vi "Spätzle_Control.vi"() -> ()   [LabVIEW 2014]
doc: "Mit diesem VI wird eine Autowäsche simuliert. Mit den Waschprogrammelementen wählen Sie die gewünschten Optionen aus. Wenn keine Option ausgewählt wird, ist die Hochdruckreinigung das Standardwaschprogramm. Nach Klick auf \"Start\" beginnt die Wäsche. Mit dem Element \"Schieberegler für Fahrzeugposition\" wird die Position des Fahrzeugs simuliert. Wenn sich das Fahrzeug in der falschen Position für das aktuelle Programm befindet, leuchtet die entsprechende Anzeige und das Fahrzeug muss bewegt werden. Die Anzeige der Waschanlage stellt den aktuellen Status des Waschprogramms dar. Mit der Schaltfläche \"Programm stoppen\" wird die Autowaschanlage sofort gestoppt."
uses:
  Controls/Options.ctl
  Controls/Simulation Position Control.ctl
  Controls/Indicators.ctl
  Controls/State Control Enum.ctl
panel:
  in  "Stopp":bool
  out "Time (s)":dbl format="%#.2g"
  out "Anzeigen der Waschanlage":T1
  in  "Plate Position":T2 scale=0.0..4.0
  out "Availability":bool
  in  "Start":bool
  in  "Optional Toppings":T3
  # "User Options"
  # "Machine Status"
  # "Simulation for Position"
  # "Use the slider to simulate the position of the transport system.\nThe slider has to be in the right position for each state to proceed."
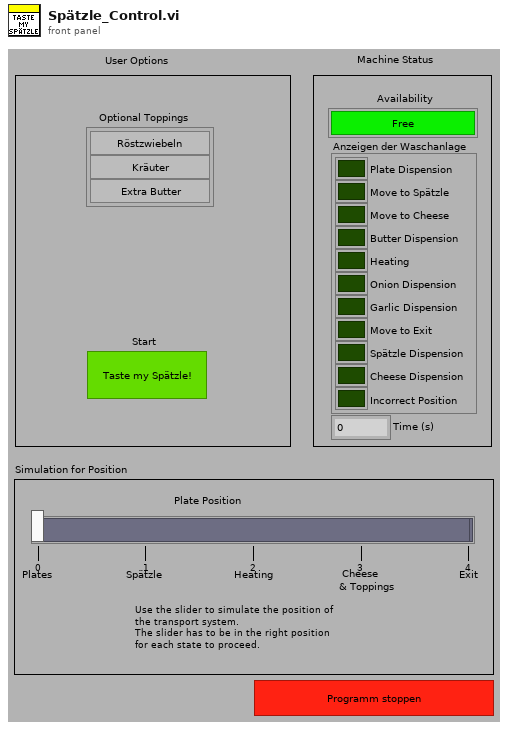
[diagram p1: front panel]
types:
  T1 = typedef "Indicators.ctl" = cluster{"Plate Dispension":bool, "Move to Spätzle":bool, "Move to Cheese":bool, "Butter Dispension":bool, "Heating":bool, "Onion Dispension":bool, "Garlic Dispension":bool, "Move to Exit":bool, "Spätzle Dispension":bool, "Cheese Dispension":bool, "Incorrect Position":bool}
  T2 = typedef "Simulation Position Control.ctl" = i32
  T3 = typedef "Options.ctl" = cluster{"Röstzwiebeln":bool, "Kräuter":bool, "Extra Butter":bool}
  T4 = typedef "State Control Enum.ctl" = enum16{"Initialize", "Wait for Start", "Plate Dispension", "Spätzle Dispension", "Heating", "Cheese Dispension", "Onion Dispension", "Garlic Dispension", "Butter Dispension", "Move to Spätzle", "Move To Cheese", "Move to Exit", "Stop", "Skip"}
  T5 = enum8{"Enabled", "Disabled", "Disabled and Grayed Out"}
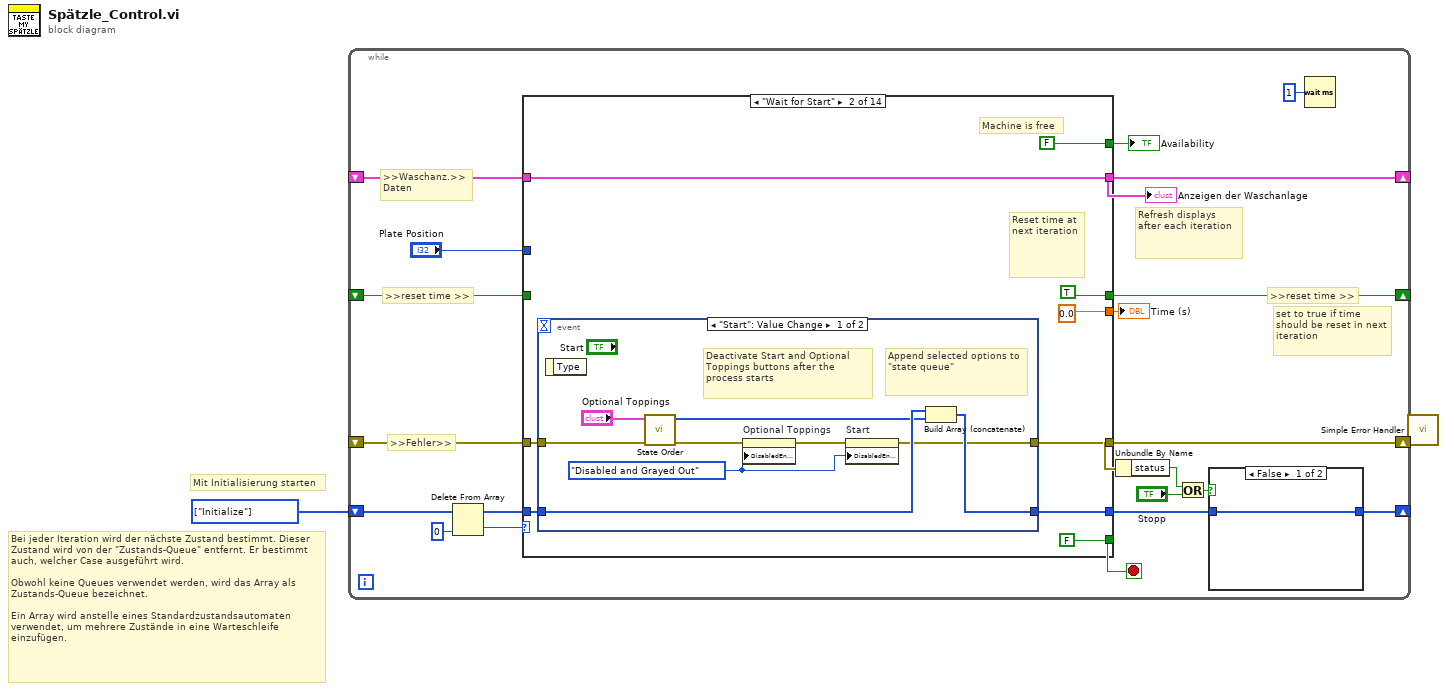
[diagram p0: block diagram]
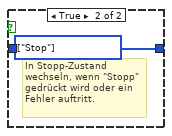
[diagram p2: hidden frame]
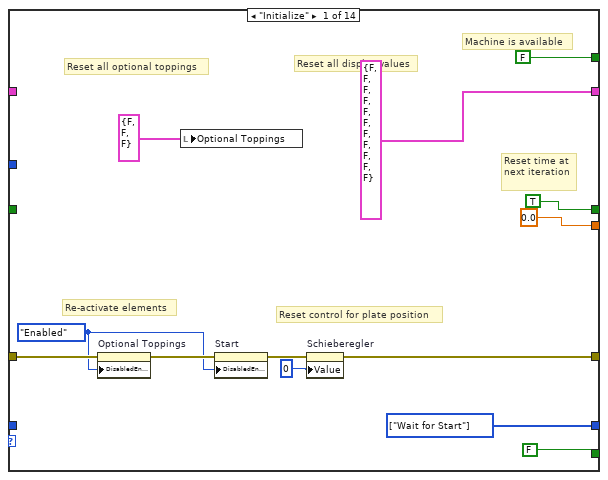
[diagram p3: hidden frame]
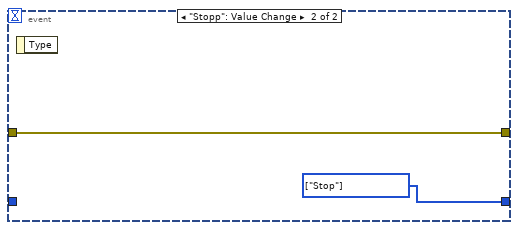
[diagram p4: hidden frame]
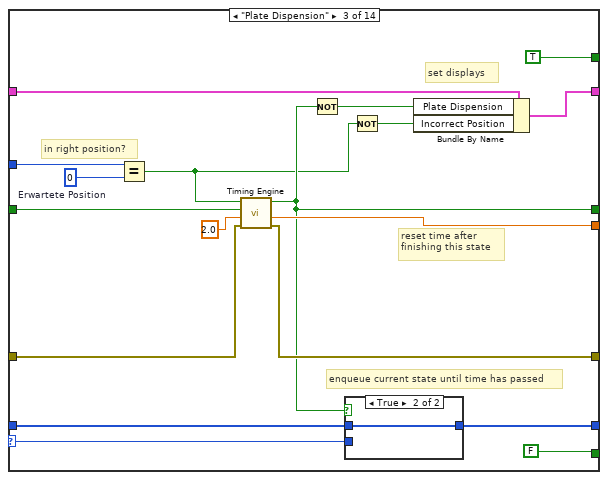
[diagram p5: hidden frame]
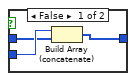
[diagram p6: hidden frame]
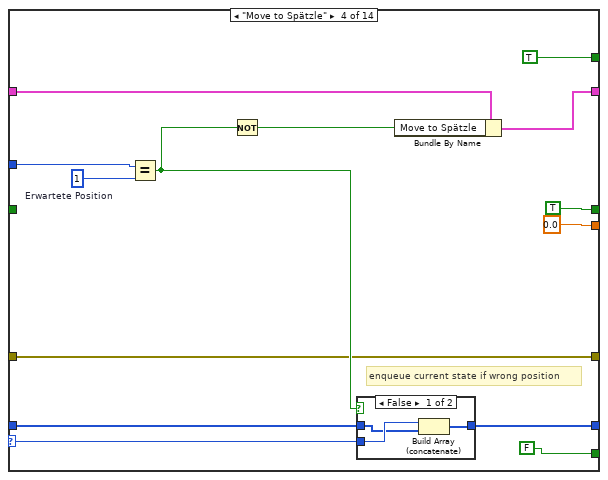
[diagram p7: hidden frame]
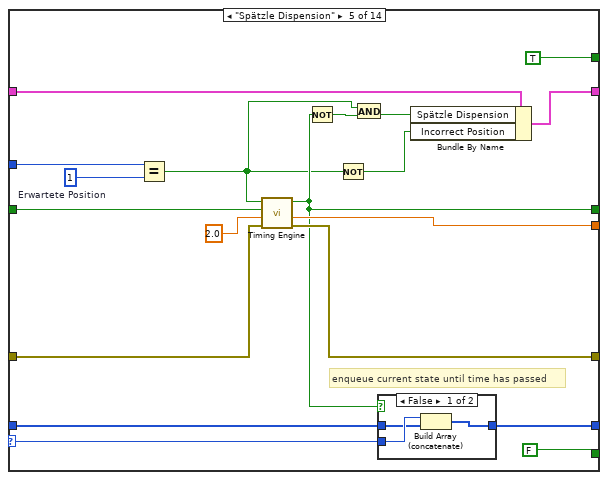
[diagram p9: hidden frame]
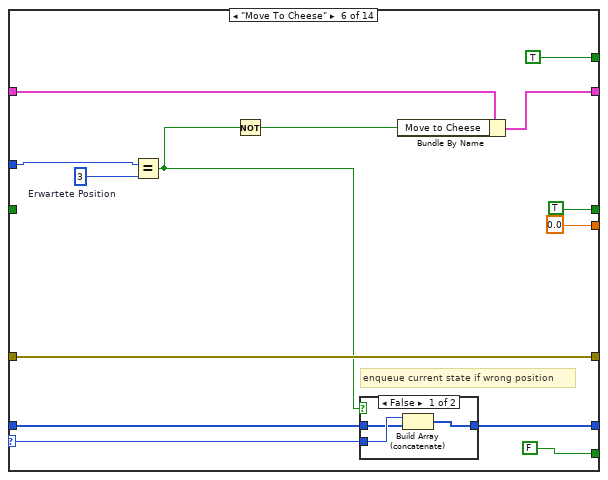
[diagram p11: hidden frame]
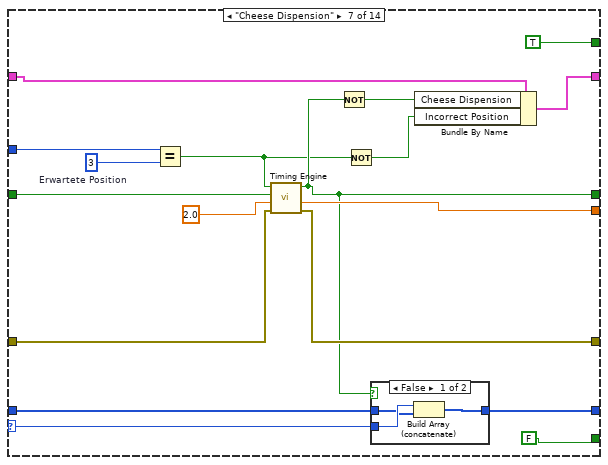
[diagram p13: hidden frame]
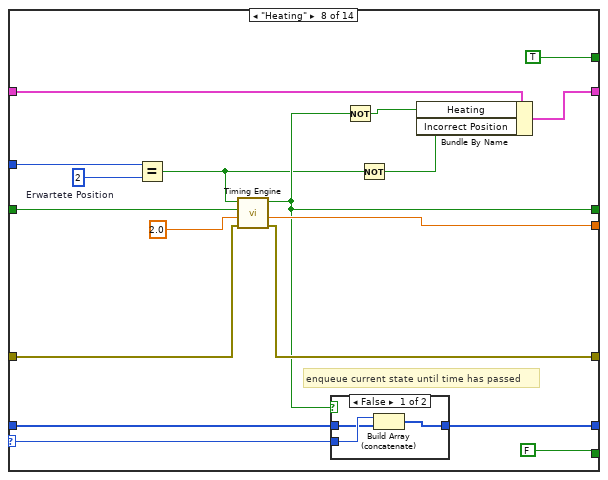
[diagram p15: hidden frame]
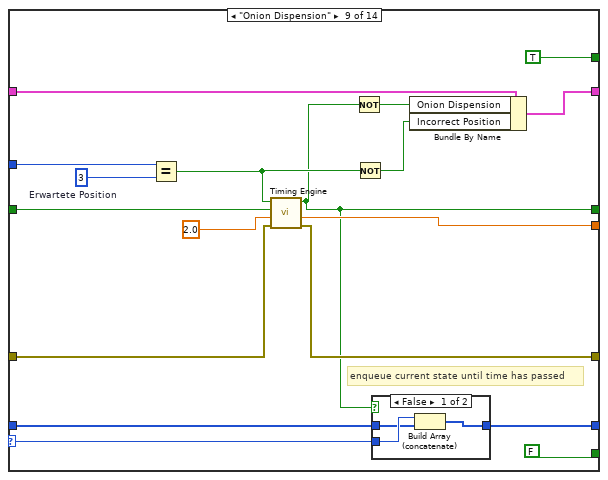
[diagram p17: hidden frame]
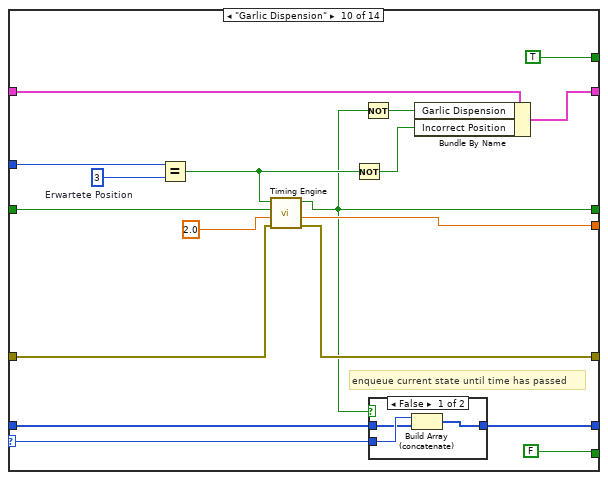
[diagram p19: hidden frame]
diagram:
  w2 = T4[] [enum."Initialize"] items=["Initialize", "Wait for Start", "Plate Dispension", "Spätzle Dispension", "Heating", "Cheese Dispension", "Onion Dispension", "Garlic Dispension", "Butter Dispension", "Move to Spätzle", "Move To Cheese", "Move to Exit", "Stop", "Skip"]
  # "Mit Initialisierung starten"
  # "Bei jeder Iteration wird der nächste Zustand bestimmt. Dieser Zustand wird von der \"Zustands-Queue\" entfernt. Er bestimmt auch, welcher Case ausgeführt wird. \n\nObwohl keine Queues verwendet werden, wird das Array als Zustands-Queue bezeichnet.  \n\nEin Array wird anstelle eines Standardzustandsautomaten verwendet, um mehrere Zustände in eine Warteschleife einzufügen."
  n1 = while "While-Schleife" {
    shift-right: [w15] -> _
    shift-left: w2 -> [w3]
    shift-right: [w18] -> _
    shift-left: _ -> [w19]
    shift-right: [w7] -> w1
    shift-left: _ -> [w14]
    shift-right: [w13] -> _
    shift-left: _ -> [w12]
    stop <- w9 stop-if-true
    # "Refresh displays after each iteration"
    # "set to true if time should be reset in next iteration"
    # ">>reset time >>"
    # ">>Fehler>>"
    # ">>Waschanz.>>\nDaten"
    # ">>reset time >>"
    n2 = Delete From Array ("Aus Array entfernen")(array=w3, index=0 ("Index")) -> (deleted portion=w20:T4, array with subset deleted=w21:T4[])  [unwired: 1 in]
    n3 = case "Case-Struktur" shown="\"Wait for Start\"" w20 {
      selector: w20 -> [_ _ w64 w83 w107 w124 w154 w170 w191 w219 w234 _ _ _]
      tunnel: w21 -> [_ w44 w63 w84 w108 w125 w153 w171 w190 w218 w233 w250 _ _]
      tunnel: [w29 w45 w65 w85 w106 w123 w152 w169 w189 w211 w235 w250 w262 w273] -> w16
      tunnel: [T1 {"Plate Dispension"=FALSE, "Move to Spätzle"=FALSE, "Move to Cheese"=FALSE, "Butter Dispension"=FALSE, "Heating"=FALSE, "Onion Dispension"=FALSE, "Garlic Dispension"=FALSE, "Move to Exit"=FALSE, "Spätzle Dispension"=FALSE, "Cheese Dispension"=FALSE, "Incorrect Position"=FALSE} ("Anzeigen der Waschanlage 2") w38 w66 w88 w109 w133 w146 w172 w192 w215 w236 w255 w266 T1 {"Plate Dispension"=FALSE, "Move to Spätzle"=FALSE, "Move to Cheese"=FALSE, "Butter Dispension"=FALSE, "Heating"=FALSE, "Onion Dispension"=FALSE, "Garlic Dispension"=FALSE, "Move to Exit"=FALSE, "Spätzle Dispension"=FALSE, "Cheese Dispension"=FALSE, "Incorrect Position"=FALSE} ("Anzeigen der Waschanlage 2")] -> w18
      tunnel: w19 -> [_ w38 w67 w89 w110 w134 w147 w173 w193 w216 w237 w255 w265 _]
      tunnel: [FALSE ("Einfahrt") FALSE ("Einfahrt") TRUE ("Einfahrt") TRUE ("Einfahrt") TRUE ("Einfahrt") TRUE ("Einfahrt") TRUE ("Einfahrt") TRUE ("Einfahrt") TRUE ("Einfahrt") TRUE ("Einfahrt") TRUE ("Einfahrt") TRUE ("Einfahrt") TRUE ("Einfahrt") FALSE ("Einfahrt")] -> w17
      tunnel: w14 -> [w35 w43 w71 w80 w112 w129 w150 w166 w197 w212 w242 w251 w261 w280]
      tunnel: [w25 w42 w72 w80 w111 w129 w151 w167 w196 w220 w241 w252 w261 w279] -> w7
      tunnel: [TRUE ("Zeit abgelaufen?") TRUE ("Einfahrt") w61 TRUE ("Zeit abgelaufen?") w103 TRUE ("Zeit abgelaufen?") w142 w164 w184 w206 w230 w254 TRUE ("Zeit abgelaufen?") TRUE ("Zeit abgelaufen?")] -> w13
      tunnel: w12 -> [_ _ w74 _ w113 _ w149 w175 w194 w213 w240 w254 _ _]
      tunnel: [0.0 ("Verstrichene Zeit") 0.0 ("Verstrichene Zeit") w73 0.0 ("Verstrichene Zeit") w104 0.0 ("Verstrichene Zeit") w145 w174 w198 w217 w238 w253 0.0 ("Verstrichene Zeit") 0.0 ("Verstrichene Zeit")] -> w11
      tunnel: "Plate Position" -> [_ _ w69 w90 w114 w127 w148 w176 w195 w214 w239 _ w268 _]
      tunnel: [FALSE ("Einfahrt") FALSE ("Einfahrt") FALSE ("Einfahrt") FALSE ("Einfahrt") FALSE ("Einfahrt") FALSE ("Einfahrt") FALSE ("Einfahrt") FALSE ("Einfahrt") FALSE ("Einfahrt") FALSE ("Einfahrt") FALSE ("Einfahrt") FALSE ("Einfahrt") FALSE ("Einfahrt") TRUE ("Einfahrt")] -> w9
      frame "Initialize" {
        w29 = T4[] [enum."Wait for Start"] items=["Initialize", "Wait for Start", "Plate Dispension", "Spätzle Dispension", "Heating", "Cheese Dispension", "Onion Dispension", "Garlic Dispension", "Butter Dispension", "Move to Spätzle", "Move To Cheese", "Move to Exit", "Stop", "Skip"]
        w26 = T5."Enabled" ("Deaktiviert")
        # "Reset time at next iteration"
        # "Re-activate elements"
        # "Reset control for plate position"
        # "Machine is available"
        # "Reset all display values"
        # "Reset all optional toppings"
        n4 = property on="Optional Toppings" class="Clust (strict)"(error in=w35, "DisabledEnum"=w26) -> (error out=w34:errorcluster)  [unwired: 1 in, 1 out]
        n5 = local write "Optional Toppings"(T3 {"Röstzwiebeln"=FALSE, "Kräuter"=FALSE, "Extra Butter"=FALSE} ("Waschprogramme")) -> ()
        n6 = property on="Start" class="Bool"(error in=w34, "DisabledEnum"=w26) -> (error out=w28:errorcluster)  [unwired: 1 in, 1 out]
        n7 = property on="Schieberegler" class="Slide (strict)"(error in=w28, "Value"=0) -> (error out=w25:errorcluster)  [unwired: 1 in, 1 out]
      }
      frame "Wait for Start" {
        # "Reset time at next iteration"
        # "Machine is free"
        n8 = event shown="[0] \"Start\": Value Change" {
          selector: _ -> [_ _]
          dyn-events: _ -> [_ _]
          timeout: _ -> [_ _]
          tunnel: [w51 w57] -> w45
          tunnel: w44 -> [w53 _]
          tunnel: [w47 w56] -> w42
          tunnel: w43 -> [w48 w56]
          event "Start": Value Change {
            w49 = T5."Disabled and Grayed Out" ("Deaktiviert")
            # "Append selected options to \"state queue\""
            # "Deactivate Start and Optional Toppings buttons after the process starts"
            n9 = event-data ("Ereignisdatenknoten")() -> ()  [unwired: 2 out]
            n10 = call "State Order.vi"("Fehler (Eingang)"=w48, "Options"="Optional Toppings") -> ("Fehler (Ausgang)"=w54:errorcluster, "States"=w52:T4[])  [unwired: 8 out]
            n11 = property on="Optional Toppings" class="Clust (strict)"(error in=w54, "DisabledEnum"=w49) -> (error out=w50:errorcluster)  [unwired: 1 in, 1 out]
            n12 = property on="Start" class="Bool"(error in=w50, "DisabledEnum"=w49) -> (error out=w47:errorcluster)  [unwired: 1 in, 1 out]
            n13 = Build Array (concatenate) ("Array erstellen")(w53, w52) -> (w51:T4[])
          }
          event "Stopp": Value Change {
            w57 = T4[] [enum."Stop"] items=["Initialize", "Wait for Start", "Plate Dispension", "Spätzle Dispension", "Heating", "Cheese Dispension", "Onion Dispension", "Garlic Dispension", "Butter Dispension", "Move to Spätzle", "Move To Cheese", "Move to Exit", "Stop", "Skip"]
            n14 = event-data ("Ereignisdatenknoten")() -> ()  [unwired: 2 out]
          }
        }
      }
      frame "Plate Dispension" {
        w68 = T2 0  # Erwartete Position
        # "in right position?"
        # "enqueue current state until time has passed"
        # "reset time after finishing this state"
        # "set displays"
        n15 = Equal? ("Gleich?")(x=w69, y=w68) -> (x = y?=w59:bool)
        n16 = call "Timing Engine.vi"("Fehler (Eingang)"=w71, "Zeitbegrenzung"=2.0 ("Waschzykluszeit"), "Zurücksetzen"=w74, "Zeitfortschritt?"=w59) -> ("Fehler (Ausgang)"=w72:errorcluster, "Verstrichene Zeit"=w73:dbl, "Zeit abgelaufen?"=w61:bool)  [unwired: 5 out]
        n17 = Not ("NICHT")(x=w61) -> (.not. x?=w60:bool)
        n18 = case shown="True" w61 {
          tunnel: [w78 w79] -> w65
          tunnel: w64 -> [w77 _]
          tunnel: w63 -> [w76 w79]
          frame False {
            n19 = Build Array (concatenate) ("Array erstellen")(w77, w76) -> (w78:T4[])
          }
          frame True {
          }
        }
        n20 = Not(x=w59) -> (.not. x?=w58:bool)
        n21 = Bundle By Name ("Nach Namen bündeln")(cluster=w67, "Plate Dispension"=w60, "Incorrect Position"=w58) -> (w66:T1)
      }
      frame "Move to Spätzle" {
        w91 = T2 1  # Erwartete Position
        # "enqueue current state if wrong position"
        n22 = Equal?(x=w90, y=w91) -> (x = y?=w92:bool)
        n23 = Not(x=w92) -> (.not. x?=w93:bool)
        n24 = case shown="False" w92 {
          tunnel: [w94 w97] -> w85
          tunnel: w84 -> [w95 w97]
          tunnel: w83 -> [w96 _]
          frame False {
            n25 = Build Array (concatenate)(w96, w95) -> (w94:T4[])
          }
          frame True {
          }
        }
        n26 = Bundle By Name ("Nach Namen bündeln")(cluster=w89, "Move to Spätzle"=w93) -> (w88:T1)
      }
      frame "Spätzle Dispension" {
        w102 = T2 1  # Erwartete Position
        # "enqueue current state until time has passed"
        n27 = Equal? ("Gleich?")(x=w114, y=w102) -> (x = y?=w98:bool)
        n28 = call "Timing Engine.vi"("Fehler (Eingang)"=w112, "Zeitbegrenzung"=2.0 ("Waschzykluszeit"), "Zurücksetzen"=w113, "Zeitfortschritt?"=w98) -> ("Fehler (Ausgang)"=w111:errorcluster, "Verstrichene Zeit"=w104:dbl, "Zeit abgelaufen?"=w103:bool)  [unwired: 5 out]
        n29 = Not ("NICHT")(x=w103) -> (.not. x?=w101:bool)
        n30 = Not(x=w98) -> (.not. x?=w100:bool)
        n31 = And(x=w98, y=w101) -> (x .and. y?=w99:bool)
        n32 = case shown="False" w103 {
          tunnel: [w119 w120] -> w106
          tunnel: w107 -> [w118 _]
          tunnel: w108 -> [w117 w120]
          frame False {
            n33 = Build Array (concatenate) ("Array erstellen")(w118, w117) -> (w119:T4[])
          }
          frame True {
          }
        }
        n34 = Bundle By Name ("Nach Namen bündeln")(cluster=w110, "Spätzle Dispension"=w99, "Incorrect Position"=w100) -> (w109:T1)
      }
      frame "Move To Cheese" {
        w126 = T2 3  # Erwartete Position
        # "enqueue current state if wrong position"
        n35 = Equal?(x=w127, y=w126) -> (x = y?=w122:bool)
        n36 = Not(x=w122) -> (.not. x?=w121:bool)
        n37 = case shown="False" w122 {
          tunnel: [w137 w138] -> w123
          tunnel: w124 -> [w136 _]
          tunnel: w125 -> [w135 w138]
          frame False {
            n38 = Build Array (concatenate) ("Array erstellen")(w136, w135) -> (w137:T4[])
          }
          frame True {
          }
        }
        n39 = Bundle By Name ("Nach Namen bündeln")(cluster=w134, "Move to Cheese"=w121) -> (w133:T1)
      }
      frame "Cheese Dispension" {
        w143 = T2 3  # Erwartete Position
        n40 = Equal? ("Gleich?")(x=w148, y=w143) -> (x = y?=w141:bool)
        n41 = call "Timing Engine.vi"("Fehler (Eingang)"=w150, "Zeitbegrenzung"=2.0 ("Waschzykluszeit"), "Zurücksetzen"=w149, "Zeitfortschritt?"=w141) -> ("Fehler (Ausgang)"=w151:errorcluster, "Verstrichene Zeit"=w145:dbl, "Zeit abgelaufen?"=w142:bool)  [unwired: 5 out]
        n42 = Not(x=w142) -> (.not. x?=w139:bool)
        n43 = Not(x=w141) -> (.not. x?=w140:bool)
        n44 = case shown="False" w142 {
          tunnel: [w159 w160] -> w152
          tunnel: w154 -> [w158 _]
          tunnel: w153 -> [w157 w160]
          frame False {
            n45 = Build Array (concatenate) ("Array erstellen")(w158, w157) -> (w159:T4[])
          }
          frame True {
          }
        }
        n46 = Bundle By Name ("Nach Namen bündeln")(cluster=w147, "Cheese Dispension"=w139, "Incorrect Position"=w140) -> (w146:T1)
      }
      frame "Heating" {
        w165 = T2 2  # Erwartete Position
        # "enqueue current state until time has passed"
        n47 = Equal? ("Gleich?")(x=w176, y=w165) -> (x = y?=w162:bool)
        n48 = call "Timing Engine.vi"("Fehler (Eingang)"=w166, "Zeitbegrenzung"=2.0 ("Waschzykluszeit"), "Zurücksetzen"=w175, "Zeitfortschritt?"=w162) -> ("Fehler (Ausgang)"=w167:errorcluster, "Verstrichene Zeit"=w174:dbl, "Zeit abgelaufen?"=w164:bool)  [unwired: 5 out]
        n49 = case shown="False" w164 {
          tunnel: [w181 w182] -> w169
          tunnel: w170 -> [w180 _]
          tunnel: w171 -> [w179 w182]
          frame False {
            n50 = Build Array (concatenate) ("Array erstellen")(w180, w179) -> (w181:T4[])
          }
          frame True {
          }
        }
        n51 = Not(x=w164) -> (.not. x?=w161:bool)
        n52 = Not(x=w162) -> (.not. x?=w163:bool)
        n53 = Bundle By Name ("Nach Namen bündeln")(cluster=w173, "Heating"=w161, "Incorrect Position"=w163) -> (w172:T1)
      }
      frame "Onion Dispension" {
        w187 = T2 3  # Erwartete Position
        # "enqueue current state until time has passed"
        n54 = Equal? ("Gleich?")(x=w195, y=w187) -> (x = y?=w186:bool)
        n55 = call "Timing Engine.vi"("Fehler (Eingang)"=w197, "Zeitbegrenzung"=2.0 ("Waschzykluszeit"), "Zurücksetzen"=w194, "Zeitfortschritt?"=w186) -> ("Fehler (Ausgang)"=w196:errorcluster, "Verstrichene Zeit"=w198:dbl, "Zeit abgelaufen?"=w184:bool)  [unwired: 5 out]
        n56 = Not(x=w184) -> (.not. x?=w183:bool)
        n57 = Not(x=w186) -> (.not. x?=w185:bool)
        n58 = case shown="False" w184 {
          tunnel: [w203 w204] -> w189
          tunnel: w191 -> [w202 _]
          tunnel: w190 -> [w201 w204]
          frame False {
            n59 = Build Array (concatenate) ("Array erstellen")(w202, w201) -> (w203:T4[])
          }
          frame True {
          }
        }
        n60 = Bundle By Name ("Nach Namen bündeln")(cluster=w193, "Onion Dispension"=w183, "Incorrect Position"=w185) -> (w192:T1)
      }
      frame "Garlic Dispension" {
        w209 = T2 3  # Erwartete Position
        # "enqueue current state until time has passed"
        n61 = Equal? ("Gleich?")(x=w214, y=w209) -> (x = y?=w208:bool)
        n62 = call "Timing Engine.vi"("Fehler (Eingang)"=w212, "Zeitbegrenzung"=2.0 ("Waschzykluszeit"), "Zurücksetzen"=w213, "Zeitfortschritt?"=w208) -> ("Fehler (Ausgang)"=w220:errorcluster, "Verstrichene Zeit"=w217:dbl, "Zeit abgelaufen?"=w206:bool)  [unwired: 5 out]
        n63 = Not(x=w208) -> (.not. x?=w207:bool)
        n64 = Not(x=w206) -> (.not. x?=w205:bool)
        n65 = case shown="False" w206 {
          tunnel: [w225 w226] -> w211
          tunnel: w219 -> [w224 _]
          tunnel: w218 -> [w223 w226]
          frame False {
            n66 = Build Array (concatenate) ("Array erstellen")(w224, w223) -> (w225:T4[])
          }
          frame True {
          }
        }
        n67 = Bundle By Name ("Nach Namen bündeln")(cluster=w216, "Garlic Dispension"=w205, "Incorrect Position"=w207) -> (w215:T1)
      }
      frame "Butter Dispension" {
        w231 = T2 3  # Erwartete Position
        # "enqueue current state until time has passed"
        n68 = Equal? ("Gleich?")(x=w239, y=w231) -> (x = y?=w228:bool)
        n69 = call "Timing Engine.vi"("Fehler (Eingang)"=w242, "Zeitbegrenzung"=2.0 ("Waschzykluszeit"), "Zurücksetzen"=w240, "Zeitfortschritt?"=w228) -> ("Fehler (Ausgang)"=w241:errorcluster, "Verstrichene Zeit"=w238:dbl, "Zeit abgelaufen?"=w230:bool)  [unwired: 5 out]
        n70 = Not(x=w228) -> (.not. x?=w227:bool)
        n71 = Not(x=w230) -> (.not. x?=w229:bool)
        n72 = case shown="False" w230 {
          tunnel: [w247 w248] -> w235
          tunnel: w234 -> [w246 _]
          tunnel: w233 -> [w245 w248]
          frame False {
            n73 = Build Array (concatenate) ("Array erstellen")(w246, w245) -> (w247:T4[])
          }
          frame True {
          }
        }
        n74 = Bundle By Name ("Nach Namen bündeln")(cluster=w237, "Butter Dispension"=w229, "Incorrect Position"=w227) -> (w236:T1)
      }
      frame "Skip" {
        w257 = 0.0  # Zeitbegrenzung
        # "Beim Überspringen sollte nur das Timing-VI aufgerufen werden, um den Zeitstempel zu aktualisieren."
        n75 = call "Timing Engine.vi"("Fehler (Eingang)"=w251, "Zeitbegrenzung"=w257, "Zurücksetzen"=w254, "Zeitfortschritt?"=FALSE) -> ("Fehler (Ausgang)"=w252:errorcluster, "Verstrichene Zeit"=w253:dbl)  [unwired: 6 out]
      }
      frame "Move to Exit" {
        w269 = T2 4  # Erwartete Position
        # "stay in this state until moved to exit - after that, go to initialization"
        n76 = Not Equal? ("Ungleich?")(x=w268, y=w269) -> (x != y?=w259:bool)
        n77 = case shown="False" w259 {
          tunnel: [w270 w271] -> w262
          frame False {
            w270 = T4[] [enum."Initialize"] items=["Initialize", "Wait for Start", "Plate Dispension", "Spätzle Dispension", "Heating", "Cheese Dispension", "Onion Dispension", "Garlic Dispension", "Butter Dispension", "Move to Spätzle", "Move To Cheese", "Move to Exit", "Stop", "Skip"]
          }
          frame True {
            w271 = T4[] [enum."Move to Exit"] items=["Initialize", "Wait for Start", "Plate Dispension", "Spätzle Dispension", "Heating", "Cheese Dispension", "Onion Dispension", "Garlic Dispension", "Butter Dispension", "Move to Spätzle", "Move To Cheese", "Move to Exit", "Stop", "Skip"]
          }
        }
        n78 = Bundle By Name ("Nach Namen bündeln")(cluster=w265, "Move to Exit"=w259, "Incorrect Position"=w259) -> (w266:T1)
      }
      frame "Stop" {
        w273 = T4[] [enum."Stop"] items=["Initialize", "Wait for Start", "Plate Dispension", "Spätzle Dispension", "Heating", "Cheese Dispension", "Onion Dispension", "Garlic Dispension", "Butter Dispension", "Move to Spätzle", "Move To Cheese", "Move to Exit", "Stop", "Skip"]
        w278 = T5."Enabled" ("Deaktiviert")
        # "reset displays"
        # "set position to start"
        # "FP-Elemente wieder aktivieren"
        n79 = local write "Plate Position"(T2 0 ("Schieberegler für Fahrzeugposition")) -> ()
        n80 = property on="Optional Toppings" class="Clust (strict)"(error in=w280, "DisabledEnum"=w278) -> (error out=w281:errorcluster)  [unwired: 1 in, 1 out]
        n81 = property on="Start" class="Bool"(error in=w281, "DisabledEnum"=w278) -> (error out=w279:errorcluster)  [unwired: 1 in, 1 out]
      }
    }
    "Anzeigen der Waschanlage" <- w18
    "Availability" <- w17
    "Time (s)" <- w11
    n82 = Unbundle By Name ("Nach Namen aufschlüsseln")(w7) -> ("status"=w6:bool)
    n83 = Or ("ODER")(x=w6, y="Stopp") -> (x .or. y?=w4:bool)
    n84 = case "Case-Struktur" shown="False" w4 {
      tunnel: w16 -> [w23 _]
      tunnel: [w23 w24] -> w15
      frame False {
      }
      frame True {
        w24 = T4[] [enum."Stop"] items=["Initialize", "Wait for Start", "Plate Dispension", "Spätzle Dispension", "Heating", "Cheese Dispension", "Onion Dispension", "Garlic Dispension", "Butter Dispension", "Move to Spätzle", "Move To Cheese", "Move to Exit", "Stop", "Skip"]
        # "In Stopp-Zustand wechseln, wenn \"Stopp\" gedrückt wird oder ein Fehler auftritt."
      }
    }
    n85 = Wait (ms) ("Warten (ms)")(milliseconds to wait=u32 1 ("Zu wartende ms")) -> ()  [unwired: 1 out]
  }
  n86 = call <vilib>:"Simple Error Handler.vi"("error in (no error)"=w1) -> ()  [unwired: 1 in, 8 out]
